vi "Write FP Control.vi"(6 "Field name":string, 8 "error in (no error)":errorcluster, 9 "Control Value":variant, 10 "Control Name":string="Configuration", 11 "Measure Object in":refnum<class "Lock-in.lvclass">) -> (0 "error out":errorcluster, 3 "Measure Object out":refnum<class "Lock-in.lvclass">)   [LabVIEW 2019, in "Lock-in.lvclass"]
uses:
  Lock-in.lvclass
  Read Lock-in Configuration.vi
  Instrument Actor/Instrument Actor.lvclass
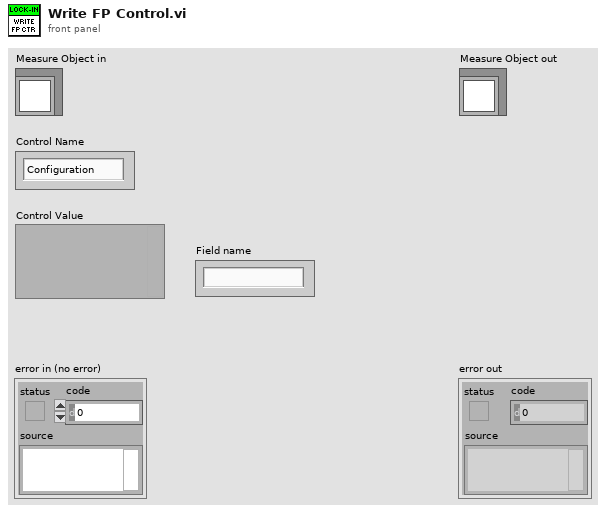
[diagram p1: front panel]
types:
  T1 = typedef "Lock-in Configuration.ctl" = cluster{"Frequency":dbl, "Time constant":dbl, "Synchronous":bool, "Channels":i32[]}
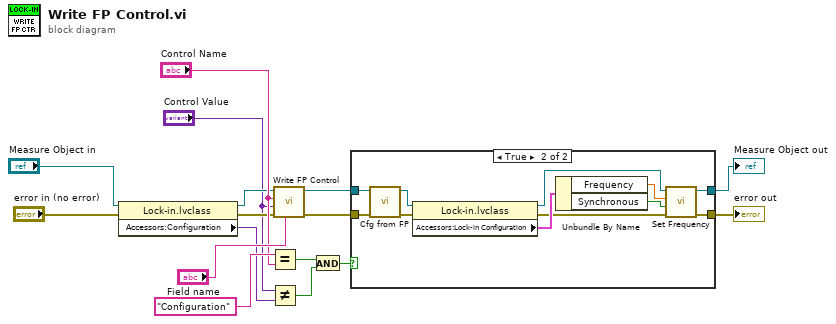
[diagram p0: block diagram]
diagram:
  n1 = property class="Lock-in.lvclass"(reference="Measure Object in", error in="error in (no error)") -> (reference out=w5:refnum<class "Lock-in.lvclass">, error out=w7:errorcluster, "Accessors:Configuration"=w3:variant)
  n2 = Equal?(x="Configuration" ("Control Name"), y="Control Name") -> (x = y?=w8:bool)
  n3 = Not Equal?(x="Control Value", y=w3) -> (x != y?=w1:bool)
  n4 = call-parent "Write FP Control.vi"("Field name"="Field name", "error in (no error)"=w7, "Control Value"="Control Value", "Control Name"="Control Name", "Measure Object in"=w5) -> ("error out"=w16:errorcluster, "Measure Object out"=w13:refnum<class "Lock-in.lvclass">)  [unwired: 5 in]
  n5 = And(x=w8, y=w1) -> (x .and. y?=w2:bool)
  n6 = case shown="True" w2 {
    tunnel: w16 -> [w17 w20]
    tunnel: w13 -> [w18 w22]
    tunnel: [w18 w27] -> w12
    tunnel: [w17 w25] -> w11
    frame False {
    }
    frame True {
      n7 = call-dynamic "Cfg from FP.vi"("error in (no error)"=w20, "Measure Object in"=w22) -> ("error out"=w19:errorcluster, "Measure Object out"=w21:refnum<class "Lock-in.lvclass">)  [unwired: 8 in]
      n8 = property class="Lock-in.lvclass"(reference=w21, error in=w19) -> (reference out=w28:refnum<class "Lock-in.lvclass">, error out=w26:errorcluster, "Accessors:Lock-in Configuration"=w29:T1)
      n9 = Unbundle By Name(w29) -> ("Frequency"=w24:dbl, "Synchronous"=w23:bool)
      n10 = call-dynamic "Set Frequency.vi"("error in (no error)"=w26, "Synchronous"=w23, "Frequency"=w24, "Lock-in in"=w28) -> ("error out"=w25:errorcluster, "Lock-in out"=w27:refnum<class "Lock-in.lvclass">)  [unwired: 6 in]
    }
  }
  "error out" <- w11
  "Measure Object out" <- w12
